vi "Q Vision_Camera FPS.vi"() -> (2 "Avg_FPS":dbl, 3 "FPS":dbl)   [LabVIEW 2016]
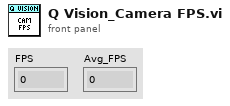
[diagram p1: front panel]
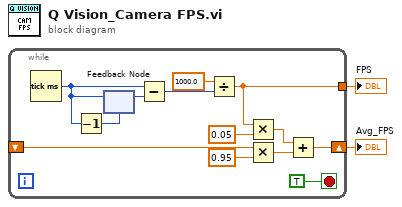
[diagram p0: block diagram]
diagram:
  n1 = while {
    tunnel: [w5] -> w2
    shift-right: [w9] -> w1
    shift-left: _ -> [w3]
    stop <- TRUE stop-if-true
    n2 = Tick Count (ms)() -> (millisecond timer value=w14:u32)
    n3 = Decrement(x=w14) -> (x-1=w4:u32)
    n4 = feedback #1(w4) -> (w15:u32)
    n5 = feedback-in #1(w14) -> ()
    n6 = Subtract(x=w14, y=w15) -> (x-y=w13:u32)
    n7 = Divide(x=1000.0 ("y"), y=w13) -> (x/y=w5:dbl)
    n8 = Multiply(x=w5, y=0.05) -> (x*y=w10:dbl)
    n9 = Multiply(x=w3, y=0.95) -> (x*y=w11:dbl)
    n10 = Add(x=w10, y=w11) -> (x+y=w9:dbl)
  }
  "FPS" <- w2
  "Avg_FPS" <- w1
